vi "LJ-T7DAQ.vi"() -> (0 "error out":errorcluster)   [LabVIEW 2015]
uses:
  CPP/InstrumentDrivers/LabJack/LabJackT7CPP-KAG/T7 IP Config KAG.ctl
  CPP/InstrumentDrivers/LabJack/LabJackT7CPP-KAG/T7 Stream Config KAG.ctl
  Globals/Meas_global.vi
  CPP/InstrumentDrivers/LabJack/LabJackT7CPP-KAG/T7 Stream Globals KAG.vi
  PWA/PWAtasksGLOBAL.vi
panel:
  in  "Path":path=path "/Macintosh HD/Users/kgompertz/Desktop/JUM Data Log/untitled"
  out "AuditTrail":string[](array[string])
  out "input terminal configuration":i32(ring)=10106 items=["default"=-1, "RSE"=10083, "NRSE"=10078, "Differential"=10106, "Pseudodifferential"=12529]
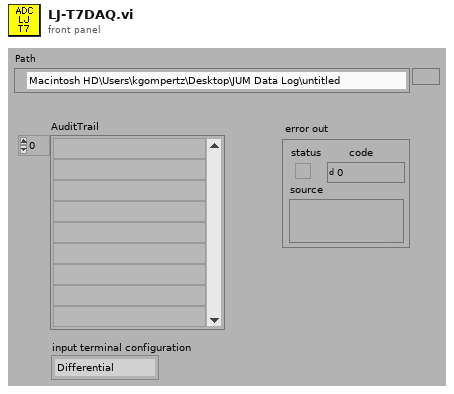
[diagram p1: front panel]
types:
  T1 = typedef "Ch_and_Spans.ctl" = cluster{"high limit (10V)":sgl, "low limit (-10V)":sgl, "Ch No":i16, "Var name":string, "Use Latest Calib":bool}
  T2 = typedef "T7 IP Config KAG.ctl" = cluster{"Connection ID In":refnum<k5>, "Connection ID Out":refnum<k5>, "Device IP":string, "Port":i32}
  T3 = typedef "T7 Stream Config KAG.ctl" = cluster{"Scan Rate (Hz)":dbl, "Samples Per Packet":u32, "Resolution Index":u32, "Buffer Size (bytes)":u32, "NumScans":u32, "Read Timeout (ms)":dbl, "Scan Table":cluster{"Channel":u32, "BipGain":u32, "Input Config":string}[]}
  T4 = cluster{"Channel":u32, "BipGain":u32, "Input Config":string}[]
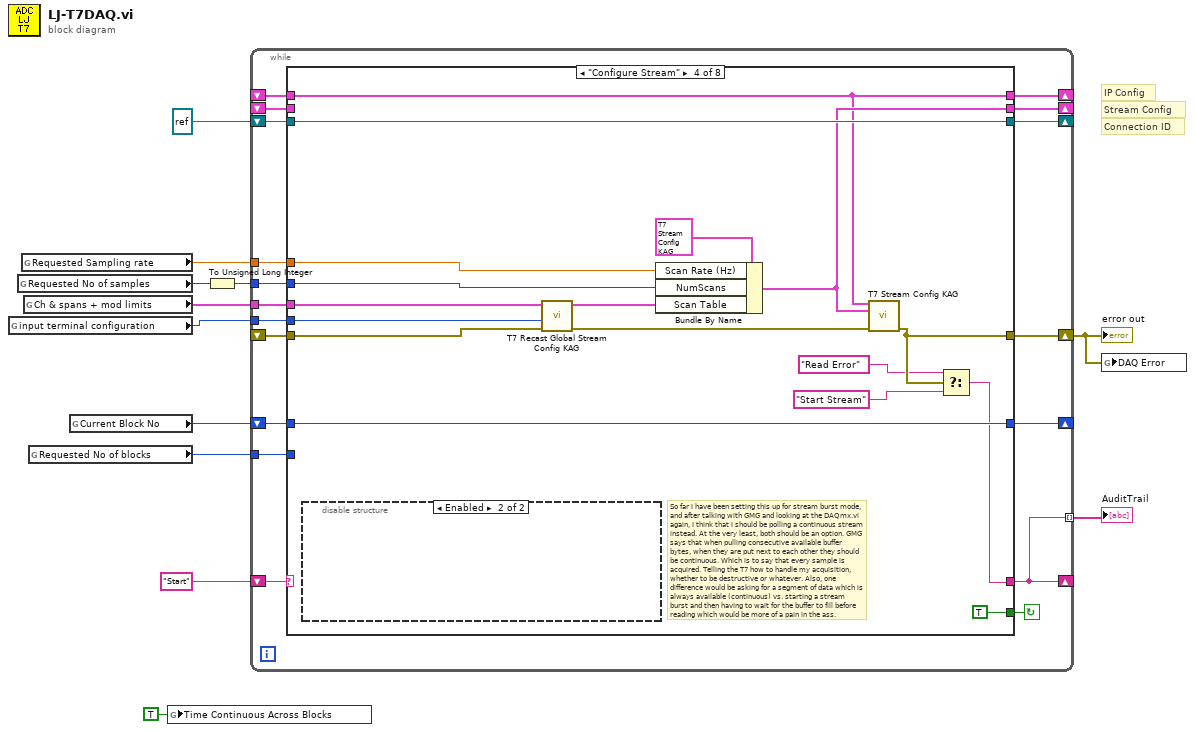
[diagram p0: block diagram]
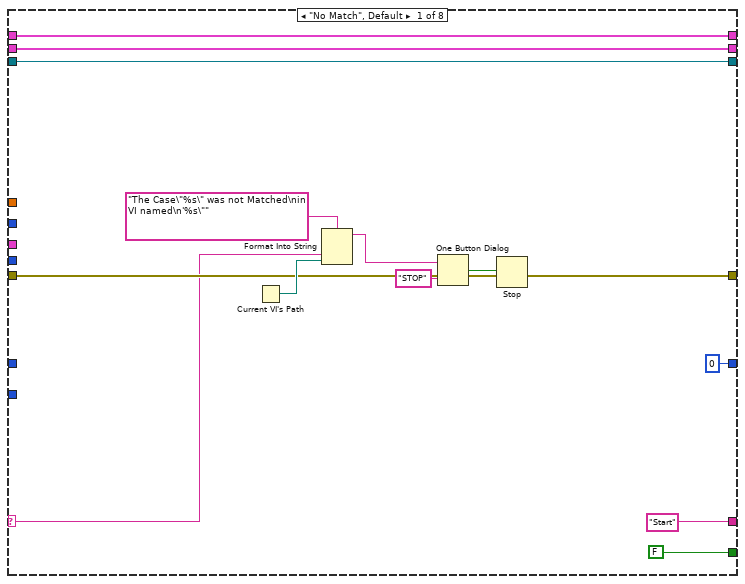
[diagram p2: hidden frame]
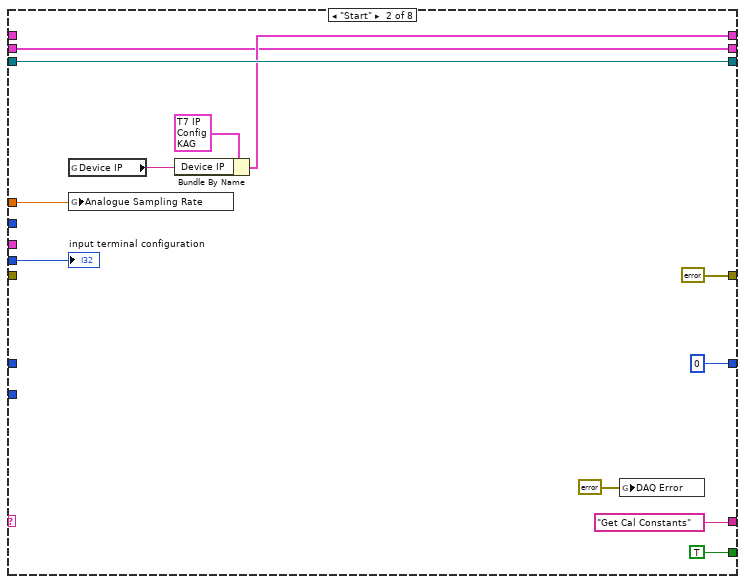
[diagram p3: hidden frame]
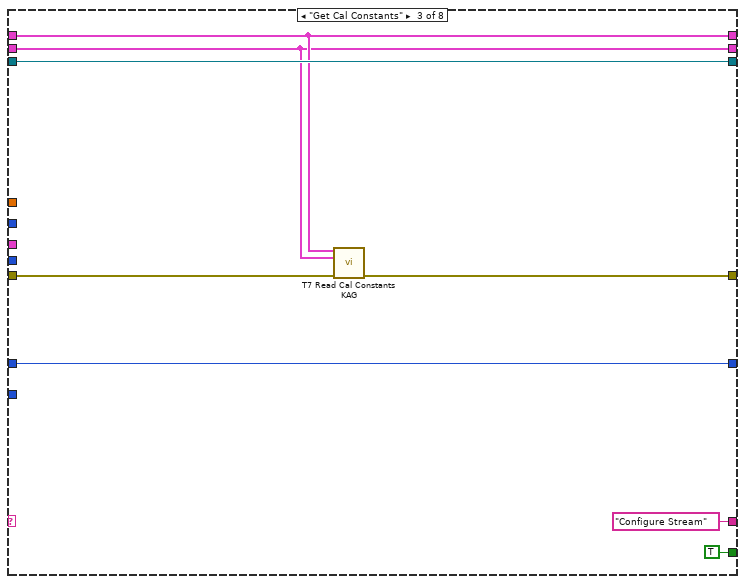
[diagram p4: hidden frame]
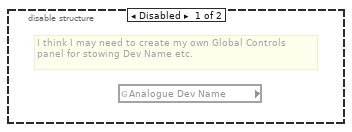
[diagram p5: hidden frame]
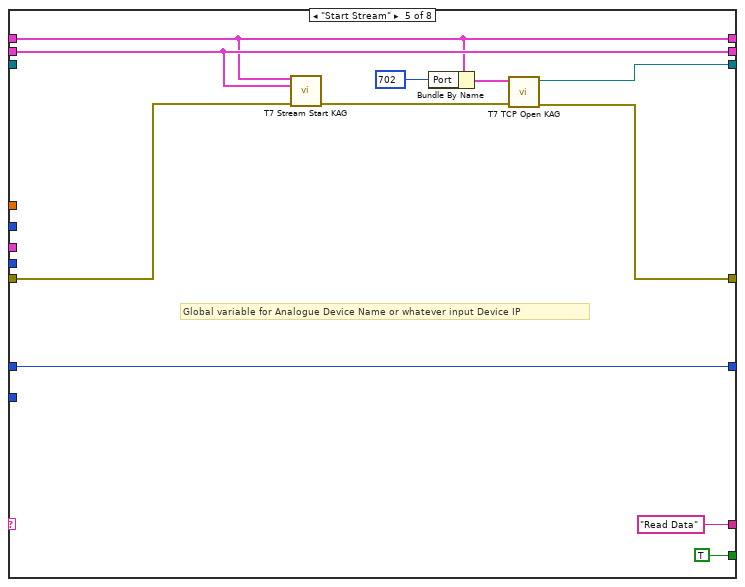
[diagram p6: hidden frame]
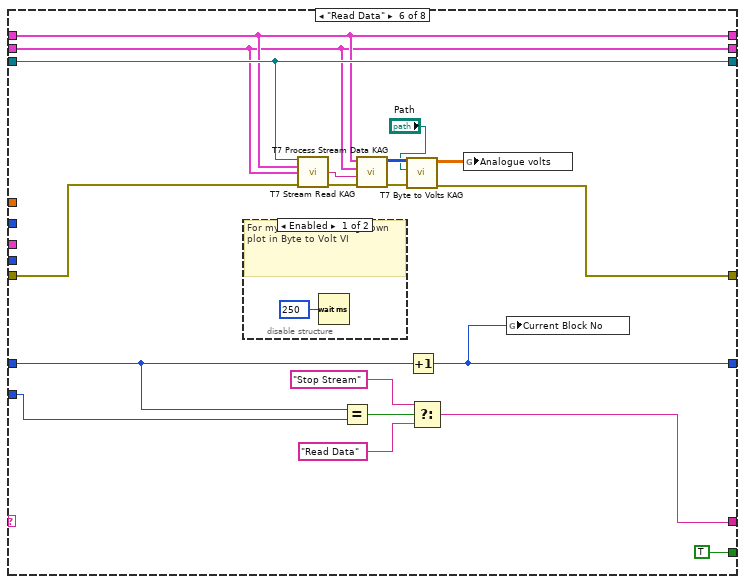
[diagram p7: hidden frame]
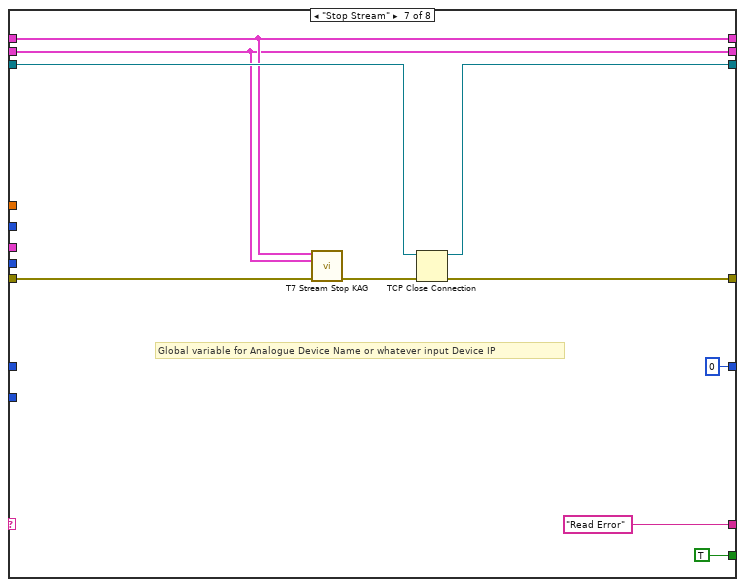
[diagram p9: hidden frame]
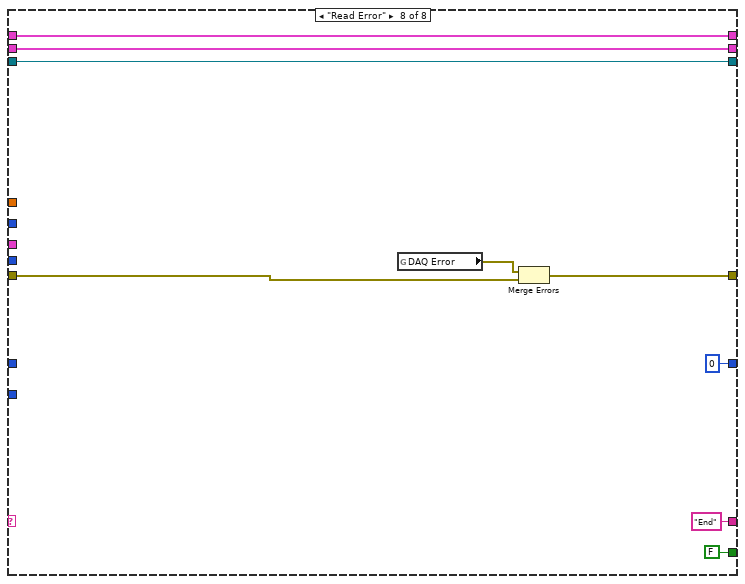
[diagram p10: hidden frame]
diagram:
  # "Connection ID"
  # "Stream Config"
  # "IP Config"
  n1 = global read "Meas_global.vi" "input terminal configuration"() -> (w1:i32)
  n2 = global read "Meas_global.vi" "Requested No of samples"() -> (w8:i32)
  n3 = global read "Meas_global.vi" "Requested Sampling rate"() -> (w7:dbl)
  n4 = global read "Meas_global.vi" "Ch & spans + mod limits"() -> (w11:T1[])
  n5 = global read "Meas_global.vi" "Requested No of blocks"() -> (w3:i32)
  n6 = global read "Meas_global.vi" "Current Block No"() -> (w10:i32)
  n7 = global write "Meas_global.vi" "Time Continuous Across Blocks"(TRUE ("Time Continuous Across Blocks")) -> ()
  n8 = To Unsigned Long Integer(number=w8) -> (unsigned 32bit integer=w6:u32)
  n9 = while {
    shift-left: "Start" -> [w29]
    shift-right: [w22] -> _
    shift-right: [w23] -> w9
    shift-left: _ -> [w28]
    tunnel: w7 -> [w27]
    tunnel: w6 -> [w26]
    tunnel: w11 -> [w24]
    tunnel: [w22] -> w5 mode=indexing
    tunnel: w3 -> [w21]
    shift-right: [w20] -> _
    shift-left: w10 -> [w25]
    shift-right: [w19] -> _
    shift-left: refnum<k5> refnum ("Connection ID Out") -> [w18]
    shift-right: [w17] -> _
    shift-left: _ -> [w16]
    shift-right: [w15] -> _
    shift-left: _ -> [w14]
    tunnel: w1 -> [w13]
    stop <- w30 continue-if-true
    n10 = case shown="\"Configure Stream\"" w29 {
      selector: w29 -> [w35 _ _ _ _ _ _ _]
      tunnel: [FALSE TRUE TRUE TRUE TRUE TRUE TRUE FALSE] -> w30
      tunnel: ["Start" "Get Cal Constants" "Configure Stream" ("f") w64 "Read Data" w100 "Read Error" "End" ("f")] -> w22
      tunnel: [w36 errorcluster {"status"=FALSE, "code"=0, "source"=""} ("error out") w62 w67 w86 w105 w114 w128] -> w23
      tunnel: w28 -> [w36 _ w63 w78 w89 w104 w119 w129]
      tunnel: w27 -> [_ w45 _ w73 _ _ _ _]
      tunnel: w26 -> [_ _ _ w72 _ _ _ _]
      tunnel: w25 -> [_ _ w59 w76 w88 w99 _ _]
      tunnel: w24 -> [_ _ _ w79 _ _ _ _]
      tunnel: w21 -> [_ _ _ _ _ w98 _ _]
      tunnel: [0 0 w59 w76 w88 w97 0 0] -> w20
      tunnel: [w33 w50 w58 w75 w85 w95 w116 w124] -> w19
      tunnel: w18 -> [w33 w50 w58 w75 _ w95 w117 w124]
      tunnel: [w32 w47 w57 w69 w81 w94 w113 w123] -> w17
      tunnel: w16 -> [w32 _ w57 w69 w81 w94 w113 w123]
      tunnel: [w31 w46 w56 w70 w82 w93 w112 w122] -> w15
      tunnel: w14 -> [w31 w46 w56 _ w82 w93 w112 w122]
      tunnel: w13 -> [_ w44 _ w68 _ _ _ _]
      frame "No Match", Default {
        n11 = Current VI's Path() -> (path=w38:path)
        n12 = Format Into String(format string="The Case\"%s\" was not Matched\nin VI named\n'%s\"" ("Format String"), w35, w38) -> (resulting string=w41:string)  [unwired: 2 in, 1 out]
        n13 = One Button Dialog(message=w41, button name ("OK")="STOP") -> (true=w39:bool)
        n14 = Stop(stop? (T)=w39) -> ()
      }
      frame "Start" {
        n15 = global read "T7 Stream Globals KAG.vi" "Device IP"() -> (w49:string)
        n16 = global write "Meas_global.vi" "Analogue Sampling Rate"(w45) -> ()
        n17 = Bundle By Name(cluster=T2 {"Connection ID In"=refnum, "Connection ID Out"=refnum, "Device IP"="192.168.126.147", "Port"=502} ("IP Configuration"), "Device IP"=w49) -> (w47:T2)
        n18 = global write "Meas_global.vi" "DAQ Error"(errorcluster {"status"=FALSE, "code"=0, "source"=""} ("DAQ Error")) -> ()
        "input terminal configuration" <- w44
      }
      frame "Get Cal Constants" {
        n19 = call "T7 Read Cal Constants KAG.vi"("IP Configuration"=w57, "Stream Configuration"=w56, "error in"=w63) -> ("error out"=w62:errorcluster)  [unwired: 11 in, 1 out]
      }
      frame "Configure Stream" {
        # "So far I have been setting this up for stream burst mode, and after talking with GMG and looking at the DAQmx.vi again, I think that I should be polling a continuous stream instead. At the very least, both should be an option. GMG says that when pulling consecutive available buffer bytes, when they are put next to each other they should be continuous. Which is to say that every sample is acquired. Telling the T7 how to handle my acquisition, whether to be destructive or whatever. Also, one difference would be asking for a segment of data which is always available (continuous) vs. starting a stream burst and then having to wait for the buffer to fill before reading which would be more of a pain in the ass."
        n20 = disable-structure shown="Enabled" {
          frame Disabled {
            # "I think I may need to create my own Global Controls panel for stowing Dev Name etc."
            n21 = global read "PWAtasksGLOBAL.vi" "Analogue Dev Name"() -> ()  [unwired: 1 out]
          }
          frame Enabled {
          }
        }
        n22 = call "T7 Recast Global Stream Config KAG.vi"("error in"=w78, "input terminal configuration"=w68, "Ch & spans + mod limits"=w79) -> ("error out"=w77:errorcluster, "Scan Table"=w71:T4)  [unwired: 3 in]
        n23 = Bundle By Name(cluster=T3 {"Scan Rate (Hz)"=1000.0, "Samples Per Packet"=512, "Resolution Index"=0, "Buffer Size (bytes)"=32768, "NumScans"=1500, "Read Timeout (ms)"=5000.0, "Scan Table"=[{"Channel"=0, "BipGain"=0, "Input Config"="Single-Ended"}, {"Channel"=1, "BipGain"=0, "Input Config"="Single-Ended"}, {"Channel"=2, "BipGain"=0, "Input Config"="Single-Ended"}, {"Channel"=3, "BipGain"=0, "Input Config"="Single-Ended"}]} ("Stream Configuration"), "Scan Rate (Hz)"=w73, "NumScans"=w72, "Scan Table"=w71) -> (w70:T3)
        n24 = call "T7 Stream Config KAG.vi"("IP Configuration"=w69, "Stream Configuration"=w70, "error in"=w77) -> ("error out"=w67:errorcluster)  [unwired: 12 in]
        n25 = Select(t="Read Error", s=w67, f="Start Stream") -> (s? t:f=w64:string)
      }
      frame "Start Stream" {
        # "Global variable for Analogue Device Name or whatever input Device IP"
        n26 = call "T7 Stream Start KAG.vi"("IP Configuration"=w81, "Stream Configuration"=w82, "error in"=w89) -> ("error out"=w87:errorcluster)  [unwired: 12 in]
        n27 = Bundle By Name(cluster=w81, "Port"=702) -> (w83:T2)
        n28 = call "T7 TCP Open KAG.vi"("error in"=w87, "IP Configuration"=w83) -> ("error out"=w86:errorcluster, "connection ID out"=w85:refnum<k5>)  [unwired: 8 in]
      }
      frame "Read Data" {
        n29 = disable-structure shown="Enabled" {
          frame Enabled {
            # "For my benefit...slowing down plot in Byte to Volt VI"
            n30 = Wait (ms)(milliseconds to wait=u32 250) -> ()  [unwired: 1 out]
          }
          frame Disabled {
          }
        }
        n31 = call "T7 Stream Read KAG.vi"("Connection ID In"=w95, "IP Configuration"=w94, "Stream Configuration"=w93, "error in"=w104) -> ("TCP Data"=w96:string, "error out"=w109:errorcluster)  [unwired: 9 in, 1 out]
        n32 = Equal?(x=w99, y=w98) -> (x = y?=w101:bool)
        n33 = call "T7 Process Stream Data KAG.vi"("error in"=w109, "TCP Data In"=w96, "Stream Configuration"=w93, "IP Configuration"=w94) -> ("error out"=w108:errorcluster, "Data"=w107:u16[][])  [unwired: 4 in, 2 out]
        n34 = call "T7 Byte to Volts KAG.vi"("error in"=w108, "file (use dialog)"="Path", "Byte Data"=w107) -> ("error out"=w105:errorcluster, "Float Data"=w106:dbl[][])  [unwired: 7 in]
        n35 = Increment(x=w99) -> (x+1=w97:i32)
        n36 = Select(t="Stop Stream", s=w101, f="Read Data") -> (s? t:f=w100:string)
        n37 = global write "Meas_global.vi" "Analogue volts"(w106) -> ()
        n38 = global write "Meas_global.vi" "Current Block No"(w97) -> ()
      }
      frame "Stop Stream" {
        # "Global variable for Analogue Device Name or whatever input Device IP"
        n39 = call "T7 Stream Stop KAG.vi"("IP Configuration"=w113, "Stream Configuration"=w112, "error in"=w119) -> ("error out"=w115:errorcluster)  [unwired: 12 in]
        n40 = TCP Close Connection(connection ID=w117, error in (no error)=w115) -> (connection ID out=w116:refnum<k5>, error out=w114:errorcluster)  [unwired: 1 in]
      }
      frame "Read Error" {
        n41 = global read "Meas_global.vi" "DAQ Error"() -> (w130:errorcluster)
        n42 = Merge Errors(w130, w129) -> (w128:errorcluster)
      }
    }
  }
  "error out" <- w9
  "AuditTrail" <- w5
  n43 = global write "Meas_global.vi" "DAQ Error"(w9) -> ()
